vi "SET.vi"(0 "refnum in":refnum<vi>, 1 "Key":string, 2 "Option":enum16{"None", "NX", "XX"}(ring), 5 "Value":string, 7 "Use EX ?":bool, 9 "Seconds":string, 11 "error in":errorcluster, 12 "Use PX ?":bool, 13 "Milliseconds":string) -> (4 "refnum out":refnum<vi>, 6 "Data":T1, 15 "error out":errorcluster)   [LabVIEW 2020]
uses:
  SubVIs/Controls/redis-data.ctl
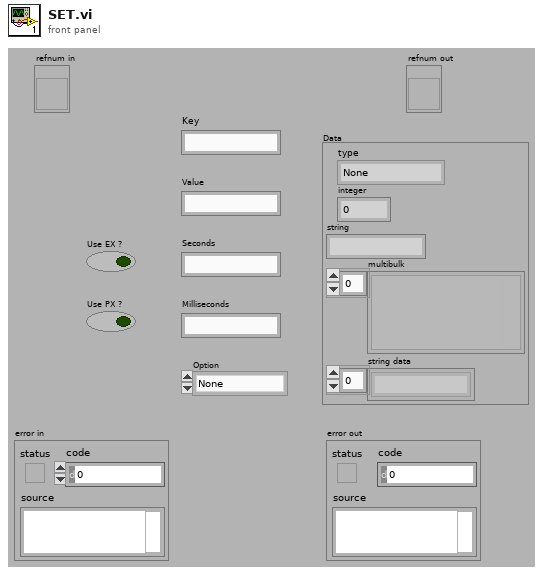
[diagram p1: front panel]
types:
  T1 = typedef "redis-data.ctl" = cluster{"type":enum16{"None", "Error", "Status", "Nil", "Integer", "String", "Multibulk"}, "integer":i64, "string":string, "multibulk":variant[], "string data":string[]}
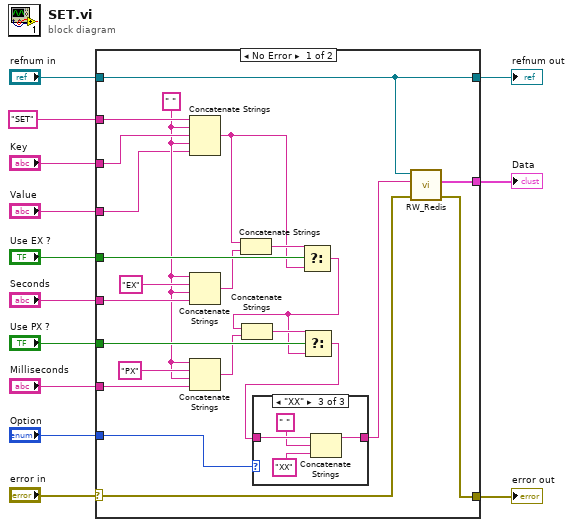
[diagram p0: block diagram]
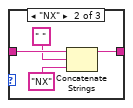
[diagram p3: hidden frame]
diagram:
  n1 = case shown="No Error" "error in" {
    selector: "error in" -> [w35 w47]
    tunnel: "Key" -> [w32 _]
    tunnel: "SET" -> [w36 _]
    tunnel: "refnum in" -> [w19 w46]
    tunnel: [w34 w47] -> w11
    tunnel: [w33 _] -> w3
    tunnel: "Seconds" -> [w31 _]
    tunnel: "Use EX ?" -> [w29 _]
    tunnel: "Use PX ?" -> [w22 _]
    tunnel: "Milliseconds" -> [w27 _]
    tunnel: [w19 w46] -> w5
    tunnel: "Value" -> [w17 _]
    tunnel: "Option" -> [w16 _]
    frame No Error {
      w18 = " "
      n2 = Concatenate Strings(w36, w18, w32, w18, w17) -> (w25:string)
      n3 = Concatenate Strings(w18, "EX", w18, w31) -> (w24:string)
      n4 = Concatenate Strings(w18, "PX", w18, w27) -> (w20:string)
      n5 = Concatenate Strings(w25, w24) -> (w26:string)
      n6 = Select(t=w26, s=w29, f=w25) -> (s? t:f=w21:string)
      n7 = Concatenate Strings(w21, w20) -> (w23:string)
      n8 = Select(t=w23, s=w22, f=w21) -> (s? t:f=w15:string)
      n9 = case shown="\"XX\"" w16 {
        tunnel: w15 -> [w37 w41 w45]
        tunnel: [w37 w38 w42] -> w14
        frame "None", Default {
        }
        frame "NX" {
          n10 = Concatenate Strings(w41, " ", "NX") -> (w38:string)
        }
        frame "XX" {
          n11 = Concatenate Strings(w45, " ", "XX") -> (w42:string)
        }
      }
      n12 = call "RW_Redis.vi"("error in"=w35, "command"=w14, "refnum"=w19) -> ("error out"=w34:errorcluster, "Data"=w33:T1)  [unwired: 7 in]
    }
    frame Error {
    }
  }
  "error out" <- w11
  "Data" <- w3
  "refnum out" <- w5
